vi "ClearAvailableRecords.vi"(8 "error in (no error)":errorcluster, 11 "Scope5761 in":refnum<class "Scope5761.lvclass">) -> (0 "error out":errorcluster, 3 "Scope5761 out":refnum<class "Scope5761.lvclass">)   [LabVIEW 2013, in "Scope5761.lvclass"]
uses:
  Scope5761.lvclass
  Scope5761.lvclass/Scope5761.ctl
  FpgaRef/FpgaRef5761/FpgaRef5761.lvclass
  FpgaRef/FpgaRef5782/FpgaRef5782.lvclass
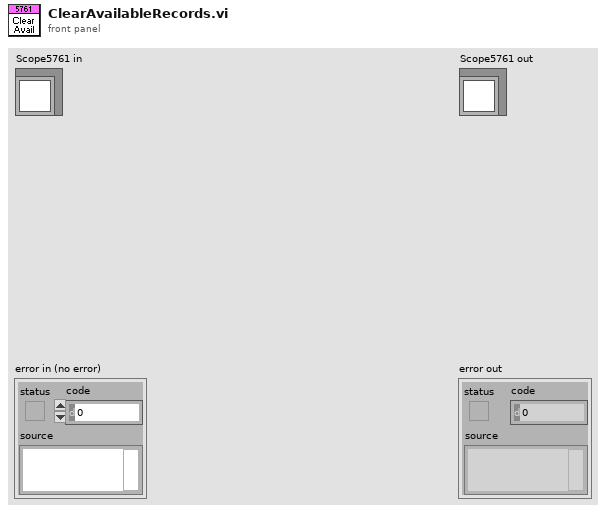
[diagram p1: front panel]
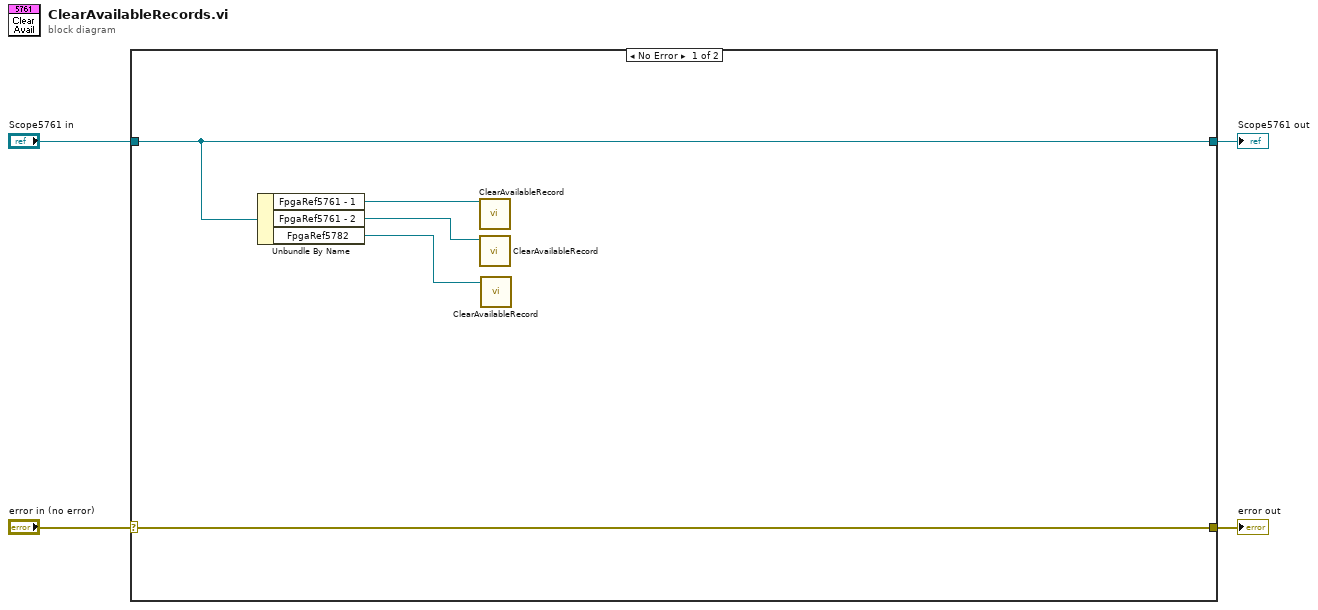
[diagram p0: block diagram]
diagram:
  n1 = case shown="No Error" "error in (no error)" {
    selector: "error in (no error)" -> [w9 w11]
    tunnel: [w9 w11] -> w3
    tunnel: [w8 w10] -> w1
    tunnel: "Scope5761 in" -> [w8 w10]
    frame No Error {
      n2 = Unbundle By Name(w8) -> ("FpgaRef5761 - 1"=w7:refnum<class "FpgaRef5761.lvclass">, "FpgaRef5761 - 2"=w6:refnum<class "FpgaRef5761.lvclass">, "FpgaRef5782"=w5:refnum<class "FpgaRef5782.lvclass">)
      n3 = call "ClearAvailableRecord.vi"("FpgaRef5761 in"=w7) -> ()  [unwired: 9 in, 2 out]
      n4 = call "ClearAvailableRecord.vi"("FpgaRef5761 in"=w6) -> ()  [unwired: 9 in, 2 out]
      n5 = call "ClearAvailableRecord.vi"("FpgaRef5782 In"=w5) -> ()  [unwired: 9 in, 2 out]
    }
    frame Error {
    }
  }
  "error out" <- w3
  "Scope5761 out" <- w1
